vi "Start Flow.vi"(6 "Enable Immediate Handshake Dispense (Disable)":bool, 7 "Address (1)":u16=1 max=15 step=1, 8 "error in (no error)":errorcluster, 9 "Number of Steps (0)":u16 max=48000 step=1, 10 "Flow Direction (0:Dispense)":u16(ring) items=["Dispense", "Aspirate", "Handshake Dispense"], 11 "VISA resource name":refnum<visa-resource-name>) -> (0 "error out":errorcluster, 1 "Busy":bool, 3 "VISA resource name out":refnum<visa-resource-name>)   [LabVIEW 2021, in "Copy of Kloehn V6 Series.lvlib"]
doc: "Uses the syringe to pump in or out fluid measured in steps. Steps can be converted to mL through the following formula:\n\n steps required = mL required\nResolution of Instrument 5000 microliters\n\nThe syringe can absorb in fluid (aspirate) or blow out fluid (dispense) or do a combination (handshake dispense). Handshake dispensing is used for multiple pumps to coordinate dispensing and aspirating."
uses:
  Copy of Kloehn V6 Series.lvlib
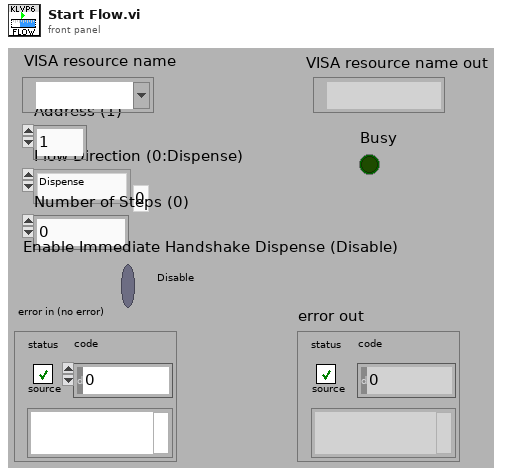
[diagram p1: front panel]
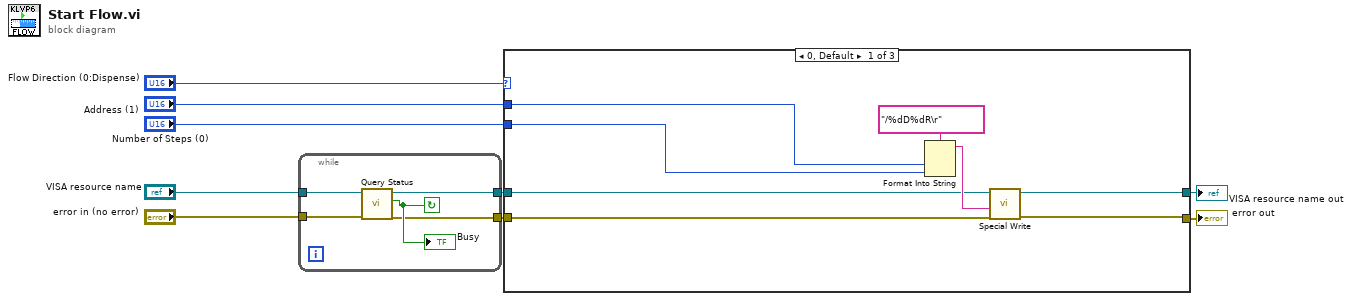
[diagram p0: block diagram]
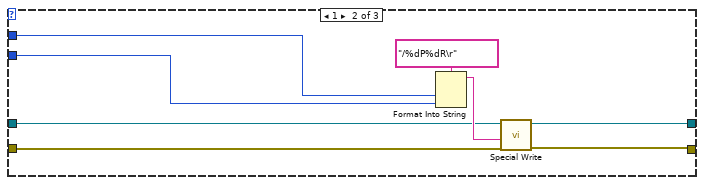
[diagram p2: hidden frame]
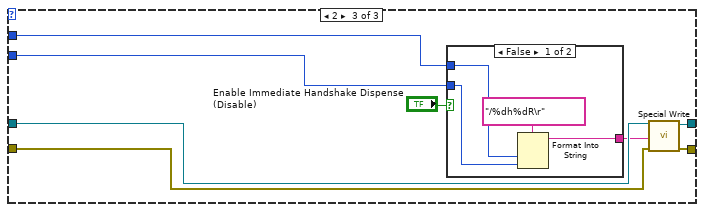
[diagram p3: hidden frame]
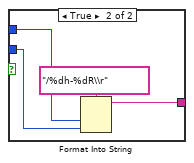
[diagram p4: hidden frame]
diagram:
  n1 = while {
    tunnel: "VISA resource name" -> [w13]
    tunnel: [w12] -> w8
    tunnel: [w11] -> w5
    tunnel: "error in (no error)" -> [w10]
    stop <- w14 continue-if-true
    n2 = call "Query Status.vi"("error in (no error)"=w10, "VISA resource name"=w13) -> ("error out"=w11:errorcluster, "Status"=w14:bool, "VISA resource name out"=w12:refnum<visa-resource-name>)  [unwired: 7 in]
    "Busy" <- w14
  }
  n3 = case shown="0, Default" "Flow Direction (0:Dispense)" {
    tunnel: "Number of Steps (0)" -> [w19 w27 w35]
    tunnel: w5 -> [w15 w25 w33]
    tunnel: w8 -> [w20 w28 w37]
    tunnel: "Address (1)" -> [w18 w26 w34]
    tunnel: [w17 w24 w31] -> w7
    tunnel: [w16 w23 w32] -> w6
    frame 0, Default {
      n4 = Format Into String(format string="/%dD%dR\r", w18, w19) -> (resulting string=w21:string)  [unwired: 2 in, 1 out]
      n5 = call "Special Write.vi"("error in (no error)"=w15, "Send String"=w21, "VISA resource name"=w20) -> ("error out"=w16:errorcluster, "VISA resource name out"=w17:refnum<visa-resource-name>)  [unwired: 4 in, 3 out]
    }
    frame 1 {
      n6 = Format Into String(format string="/%dP%dR\r", w26, w27) -> (resulting string=w30:string)  [unwired: 2 in, 1 out]
      n7 = call "Special Write.vi"("error in (no error)"=w25, "Send String"=w30, "VISA resource name"=w28) -> ("error out"=w23:errorcluster, "VISA resource name out"=w24:refnum<visa-resource-name>)  [unwired: 4 in, 3 out]
    }
    frame 2 {
      n8 = case shown="False" "Enable Immediate Handshake Dispense (Disable)" {
        tunnel: [w41 w45] -> w36
        tunnel: w35 -> [w40 w43]
        tunnel: w34 -> [w39 w44]
        frame False {
          n9 = Format Into String(format string="/%dh%dR\r", w39, w40) -> (resulting string=w41:string)  [unwired: 2 in, 1 out]
        }
        frame True {
          n10 = Format Into String(format string="/%dh-%dR\\r", w44, w43) -> (resulting string=w45:string)  [unwired: 2 in, 1 out]
        }
      }
      n11 = call "Special Write.vi"("error in (no error)"=w33, "Send String"=w36, "VISA resource name"=w37) -> ("error out"=w32:errorcluster, "VISA resource name out"=w31:refnum<visa-resource-name>)  [unwired: 4 in, 3 out]
    }
  }
  "error out" <- w6
  "VISA resource name out" <- w7
